vi "N5746A_Close.vi"(8 "error":errorcluster, 11 "VISA name":refnum<visa-resource-name>) -> (0 "error out":errorcluster)   [LabVIEW 2015]
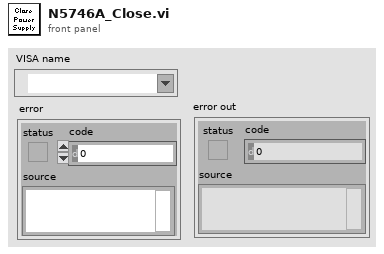
[diagram p1: front panel]
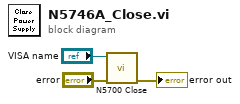
[diagram p0: block diagram]
diagram:
  n1 = call <instrlib>:"N5700 Close.vi"("error"="error", "VISA name"="VISA name") -> ("error out"=→"error out":errorcluster)  [unwired: 6 in]
